vi "checkBeginKickPenaltyAllyPlayVSS.vi"(8 "error in (no error)":errorcluster, 10 "queue 2":T1(array[ring]), 11 "KickPenaltyAllyPlayVSS in":refnum<class "KickPenaltyAllyPlayVSS.lvclass">) -> (0 "error out":errorcluster, 2 "logical AND":bool, 3 "KickPenaltyAllyPlayVSS out":refnum<class "KickPenaltyAllyPlayVSS.lvclass">)   [LabVIEW 2020, in "KickPenaltyAllyPlayVSS.lvclass"]
uses:
  KickPenaltyAllyPlayVSS.lvclass
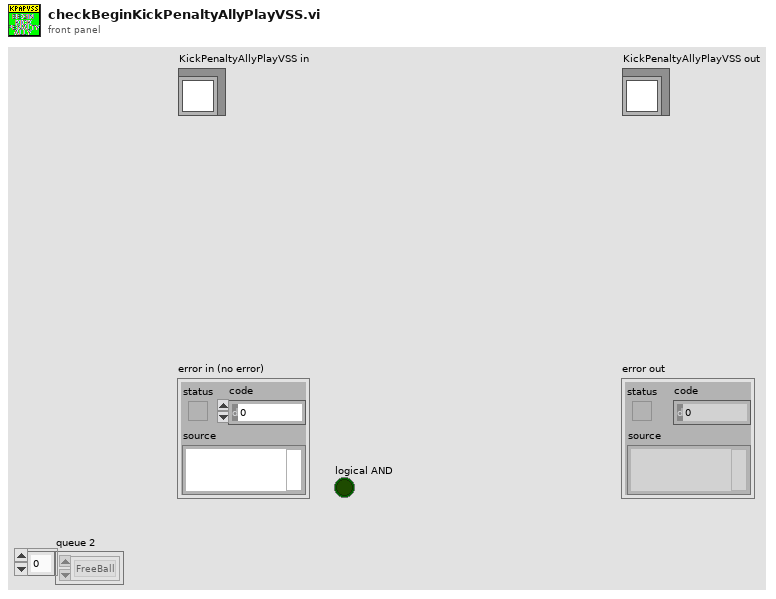
[diagram p1: front panel]
types:
  T1 = enum16{"FreeBall", "PrepareFreeBall", "GoalKickEnemy", "GoalKickAlly", "KickoffAlly", "KickoffEnemy", "PrepareGoalKickEnemy", "PrepareGoalKickAlly", "Stop", "PrepareKickoffEnemy", "PrepareKickoffAlly", "PreparePenaltyEnemy", "Timeout", "DeadBall", "NormalGame", "KickPenaltyAlly", "PenaltyEnemy", "BallChallenge", "PreparePenaltyAlly", "Halt"}[]
  T2 = enum16{"FreeBall", "PrepareFreeBall", "GoalKickEnemy", "GoalKickAlly", "KickoffAlly", "KickoffEnemy", "PrepareGoalKickEnemy", "PrepareGoalKickAlly", "Stop", "PrepareKickoffEnemy", "PrepareKickoffAlly", "PreparePenaltyEnemy", "Timeout", "DeadBall", "NormalGame", "KickPenaltyAlly", "PenaltyEnemy", "BallChallenge", "PreparePenaltyAlly", "Halt"}
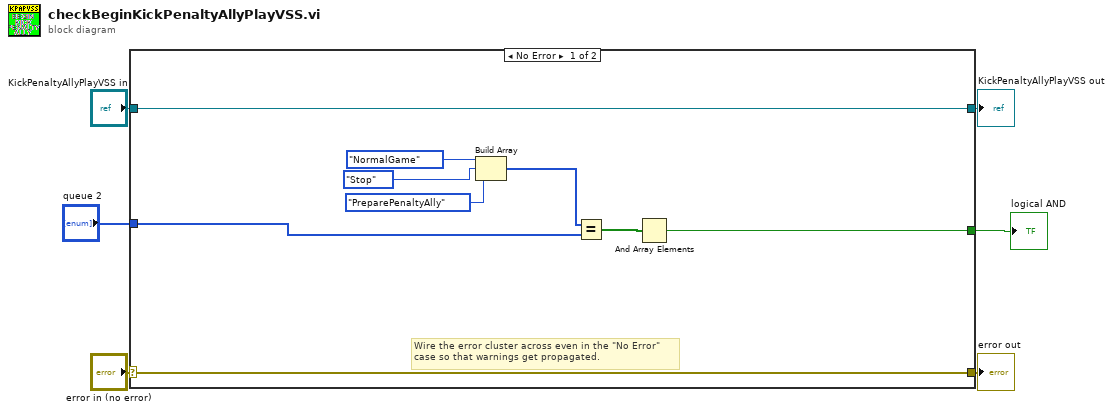
[diagram p0: block diagram]
diagram:
  n1 = case shown="No Error" "error in (no error)" {
    selector: "error in (no error)" -> [w14 w17]
    tunnel: [w14 w17] -> w5
    tunnel: [w15 w16] -> w3
    tunnel: "KickPenaltyAllyPlayVSS in" -> [w15 w16]
    tunnel: "queue 2" -> [w8 _]
    tunnel: [w7 _] -> w1
    frame No Error {
      # "Wire the error cluster across even in the \"No Error\"\ncase so that warnings get propagated."
      n2 = Build Array(T2."NormalGame" ("VssPlay"), T2."Stop" ("VssPlay"), T2."PreparePenaltyAlly" ("VssPlay")) -> (w10:T1)
      n3 = Equal?(x=w10, y=w8) -> (x = y?=w9:bool[])
      n4 = And Array Elements(Boolean array=w9) -> (logical AND=w7:bool)
    }
    frame Error {
    }
  }
  "error out" <- w5
  "KickPenaltyAllyPlayVSS out" <- w3
  "logical AND" <- w1
